vi "MaxiGauge_Status.vi"() -> (1 "n_ng":u8, 2 "values":T1)   [LabVIEW 2019]
uses:
  MaxiGauge_Global.vi
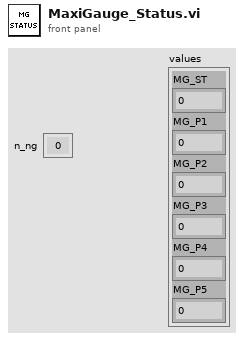
[diagram p1: front panel]
types:
  T1 = cluster{"MG_ST":u32, "MG_P1":dbl, "MG_P2":dbl, "MG_P3":dbl, "MG_P4":dbl, "MG_P5":dbl}
  T2 = enum32{"Bad", "Idle", "Run top level", "Running"}
  T3 = cluster{"MKS670_1000_ST":u32, "MG_P1":dbl, "MG_P2":dbl, "MG_P3":dbl, "MG_P4":dbl, "MG_P5":dbl}
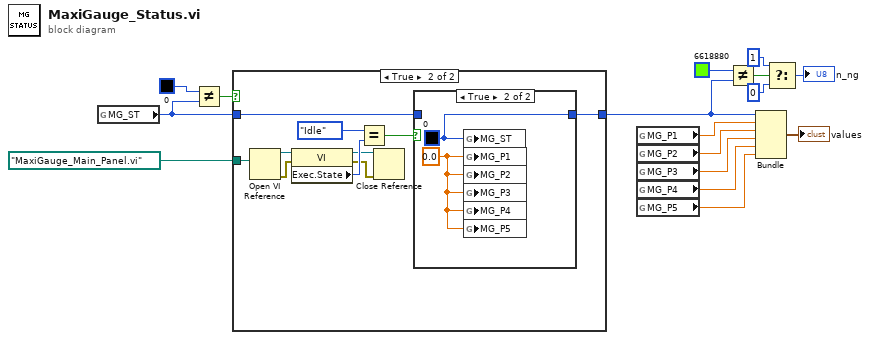
[diagram p0: block diagram]
diagram:
  n1 = global read "MaxiGauge_Global.vi" "MG_ST"() -> (w7:u32)
  n2 = Not Equal?(x=u32 0 ("MKS670_1000_ST 2"), y=w7) -> (x != y?=w16:bool)
  n3 = case shown="True" w16 {
    tunnel: w7 -> [w17 w19]
    tunnel: [w17 w18] -> w13
    tunnel: path "MaxiGauge_Main_Panel.vi" ("vi path") -> [_ w20]
    frame False {
    }
    frame True {
      n4 = Open VI Reference(vi path=w20) -> (vi reference=w27:refnum<vi>, error out=w26:errorcluster)  [unwired: 5 in]
      n5 = property class="VI"(reference=w27, error in=w26) -> (reference out=w22:refnum<vi>, error out=w21:errorcluster, "Exec.State"=w24:T2)
      n6 = Equal?(x=T2."Idle" ("Execution:State"), y=w24) -> (x = y?=w25:bool)
      n7 = Close Reference(reference=w22, error in (no error)=w21) -> ()  [unwired: 1 out]
      n8 = case shown="True" w25 {
        tunnel: w19 -> [w28 _]
        tunnel: [w28 w30] -> w18
        frame False {
        }
        frame True {
          w29 = 0.0 ("MKS670_1000_P")
          w30 = u32 0 ("MKS670_1000_ST")
          n9 = global write "MaxiGauge_Global.vi" "MG_ST"(w30) -> ()
          n10 = global write "MaxiGauge_Global.vi" "MG_P1"(w29) -> ()
          n11 = global write "MaxiGauge_Global.vi" "MG_P2"(w29) -> ()
          n12 = global write "MaxiGauge_Global.vi" "MG_P3"(w29) -> ()
          n13 = global write "MaxiGauge_Global.vi" "MG_P4"(w29) -> ()
          n14 = global write "MaxiGauge_Global.vi" "MG_P5"(w29) -> ()
        }
      }
    }
  }
  n15 = global read "MaxiGauge_Global.vi" "MG_P1"() -> (w6:dbl)
  n16 = global read "MaxiGauge_Global.vi" "MG_P2"() -> (w5:dbl)
  n17 = global read "MaxiGauge_Global.vi" "MG_P3"() -> (w2:dbl)
  n18 = global read "MaxiGauge_Global.vi" "MG_P4"() -> (w3:dbl)
  n19 = global read "MaxiGauge_Global.vi" "MG_P5"() -> (w4:dbl)
  n20 = Not Equal?(x=u32 6618880 ("MKS670_1000_ST 2"), y=w13) -> (x != y?=w11:bool)
  n21 = Bundle("MKS670_1000_ST"=w13, "MG_P1"=w6, "MG_P2"=w5, "MG_P3"=w2, "MG_P4"=w3, "MG_P5"=w4) -> (→"values":T3)  [unwired: 1 in]
  n22 = Select(t=u8 1 ("n_ng"), s=w11, f=u8 0 ("n_ng")) -> (s? t:f=→"n_ng":u8)
